vi "Define connected axes.vi"(0 "System no.":i32=1 min=1 max=4 step=1, 2 "Read from\ncontroller?":bool, 3 "Invert\norder?":bool, 4 "Conn. axes":string[](array[string]), 5 "error in":errorcluster) -> (14 "Conn. Axes out":string[](array[string]), 19 "error out":errorcluster)   [LabVIEW 2026]
doc: "Writes connected axes into Global2 (Array).vi. This VI is called automatically by PI_GCS2_Configuration_Setup.vi and must be completed successfully before any other axis-specific command VI is called. Requires SAI?.vi to be present.\n\nAnalog: Only supported when called by Analog_Configuration_Setup.vi\n\nC-702: Read from controller = TRUE, Invert order = TRUE\n\nC-848: Read from controller = TRUE, Invert order = TRUE\n\nC-880: Read from controller = TRUE, Invert order = TRUE \n\nC-887, F-206, M-8X0: Read from controller = FALSE, Invert order = FALSE, Connected axes = X,Y,Z,U,V,W, (A,B,K,L,M optional)\n\nAll other systems: Read from controller = TRUE, Invert order = FALSE"
uses:
  Global2 (Array).vi
panel:
  # "Define connected axes and write identifier into global2 (array).vi"
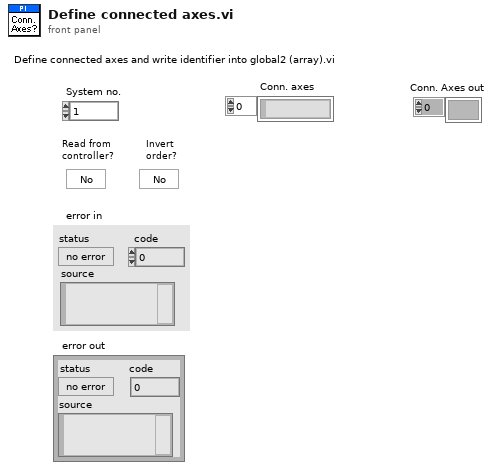
[diagram p1: front panel]
types:
  T1 = typedef "Controller names.ctl" = enum16{"None", "Analog", "C-702", "C-413", "C-414", "C-843", "C-843.PM", "C-844", "C-848", "C-865", "C-866", "C-867", "C-877", "C-880", "C-884", "C-885", "C-886", "C-887", "C-891", "E-135", "E-516", "E-517", "E-518", "E-709", "E-710", "E-712", "E-725", "E-727", "E-753", "E-754", "E-755", "E-761", "E-816", "E-861", "E-870", "E-871", "E-872", "E-873", "E-874", "F-206", "HydraPollux", "M-840", "M-850", "M-8X0", "Mercury", "Mercury_GCS", "PI_GCS2"}
  T2 = cluster{"Conn. axes":string[], "Controller name":T1}[]
  T3 = cluster{"Conn. axes":string[], "Controller name":T1}
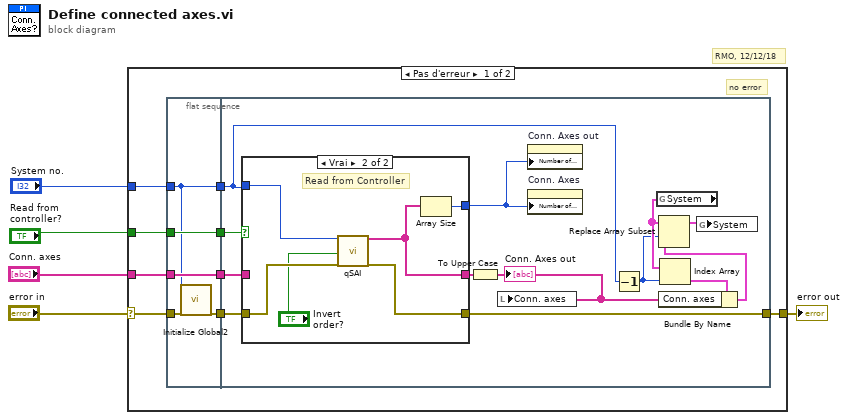
[diagram p0: block diagram]
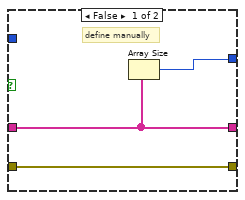
[diagram p2: hidden frame]
diagram:
  # "RMO, 12/12/18"
  n1 = case shown="Pas d'erreur" "error in" {
    selector: "error in" -> [w6 w42]
    tunnel: [w14 w42] -> w5
    tunnel: "Read from\ncontroller?" -> [w13 _]
    tunnel: "System no." -> [w11 _]
    tunnel: "Conn. axes" -> [w12 _]
    frame No Error {
      # "no error"
      n2 = flat-sequence {
        tunnel: w11 -> [w15]
        tunnel: w12 -> [w18]
        tunnel: w6 -> [w17]
        tunnel: w13 -> [w19]
        tunnel: [w19] -> w10
        tunnel: [w18] -> w9
        tunnel: [w15] -> w8
        tunnel: [w16] -> w7
        tunnel: [w32] -> w14
        tunnel: w10 -> [w31]
        tunnel: w7 -> [w30]
        tunnel: w9 -> [w29]
        tunnel: w8 -> [w25]
        frame #0 {
          n3 = call "Initialize Global2.vi"("System no."=w15, "error in"=w17) -> ("error out"=w16:errorcluster)  [unwired: 17 out]
        }
        frame #1 {
          n4 = case shown="Vrai" w31 {
            tunnel: w25 -> [_ w41]
            tunnel: w30 -> [w35 w40]
            tunnel: [w35 w39] -> w32
            tunnel: [w34 w38] -> w27
            tunnel: w29 -> [w33 _]
            tunnel: [w33 w36] -> w28
            frame False {
              # "define manually"
              n5 = Array Size(array=w33) -> (size(s)=w34:i32)
            }
            frame True {
              # "Read from Controller"
              n6 = call "qSAI.vi"("System no."=w41, "Invert order?"="Invert\norder?", "error in"=w40) -> ("Conn. axes"=w36:string[], "error out"=w39:errorcluster)  [unwired: 3 in, 12 out]
              n7 = Array Size(array=w36) -> (size(s)=w38:i32)
            }
          }
          n8 = To Upper Case(1:w28) -> (0:w21:string[])
          "Conn. Axes out" <- w21
          n9 = local write "Conn. axes"(w21) -> ()
          n10 = property on="Conn. Axes out" class="Tabl (strict)"("Number of Rows"=w27) -> ()  [unwired: 2 in, 2 out]
          n11 = property on="Conn. Axes" class="Tabl (strict)"("Number of Rows"=w27) -> ()  [unwired: 2 in, 2 out]
          n12 = Decrement(x=w25) -> (x-1=w22:i32)
          n13 = global read "Global2 (Array).vi" "System"() -> (w23:T2)
          n14 = Index Array(array=w23, index=w22) -> (element=w24:T3)
          n15 = Bundle By Name(cluster=w24, "Conn. axes"=w21) -> (w20:T3)
          n16 = Replace Array Subset(array=w23, new element=w20, index=w22) -> (w26:T2)
          n17 = global write "Global2 (Array).vi" "System"(w26) -> ()
        }
      }
    }
    frame Error {
    }
  }
  "error out" <- w5
